vi "MeasureExportStrings.vi"() -> ()   [LabVIEW 2013]
panel:
  out "MeasureExportStrings":string[](array[string])
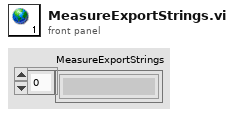
[diagram p1: front panel]
diagram:
